vi "坐标旋转-dtXY.vi"(9 "旋转角度(单位角度)":dbl, 11 "dtx,dty In":T1 {"X" format="%#.3f"}) -> (3 "dtx,dty Out":T1 {"X" format="%#.3f"})   [LabVIEW 2014]
uses:
  Controls/XYPos.ctl
panel:
  out "cos(x)":dbl
  out "sin(x)":dbl
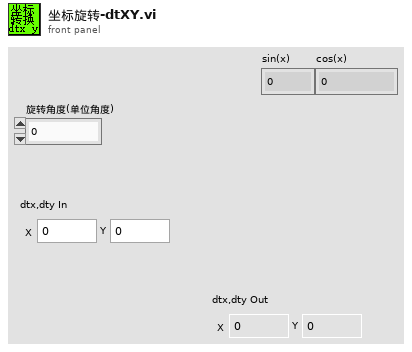
[diagram p1: front panel]
types:
  T1 = typedef "XYPos.ctl" = cluster{"X":dbl, "Y":dbl}
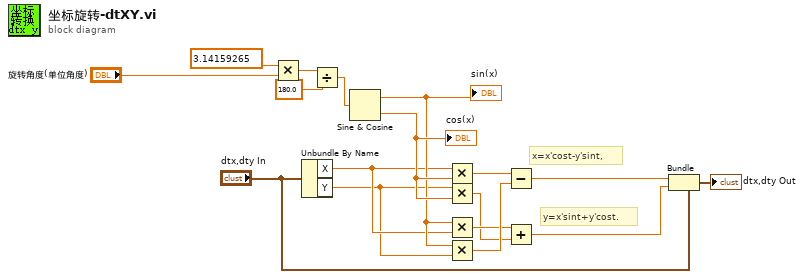
[diagram p0: block diagram]
diagram:
  # "y=x'sint+y'cost."
  # "x=x'cost-y'sint,"
  n1 = Multiply(x=3.14159265, y="旋转角度(单位角度)") -> (x*y=w3:dbl)
  n2 = Unbundle By Name("dtx,dty In") -> ("X"=w15:dbl, "Y"=w14:dbl)
  n3 = Divide(x=w3, y=180.0) -> (x/y=w2:dbl)
  n4 = Sine & Cosine(0:w2) -> (1:w16:dbl, 2:w17:dbl)
  "sin(x)" <- w16
  "cos(x)" <- w17
  n5 = Multiply(x=w15, y=w17) -> (x*y=w13:dbl)
  n6 = Multiply(x=w14, y=w17) -> (x*y=w10:dbl)
  n7 = Multiply(x=w16, y=w15) -> (x*y=w11:dbl)
  n8 = Multiply(x=w16, y=w14) -> (x*y=w12:dbl)
  n9 = Subtract(x=w13, y=w12) -> (x-y=w9:dbl)
  n10 = Add(x=w11, y=w10) -> (x+y=w8:dbl)
  n11 = Bundle(cluster="dtx,dty In", "X"=w9, "Y"=w8) -> (→"dtx,dty Out":T1)
